vi "Przeliczanie kąta na azymut.vi"(4 "Kąt [stoponie]":dbl) -> (1 "Azymut [stopnie]":dbl)   [LabVIEW 2015, in "Biblioteka moduł map v3.lvlib" / "Matematyczne.lvlib"]
uses:
  Matematyczne.lvlib
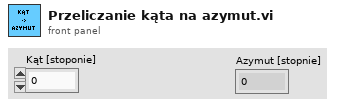
[diagram p1: front panel]
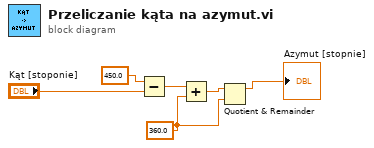
[diagram p0: block diagram]
diagram:
  w4 = 360.0 ("y")
  n1 = Subtract(x=450.0, y="Kąt [stoponie]") -> (x-y=w2:dbl)
  n2 = Add(x=w2, y=w4) -> (x+y=w5:dbl)
  n3 = Quotient & Remainder(x=w5, y=w4) -> (x-y*floor(x/y)=→"Azymut [stopnie]":dbl)  [unwired: 1 out]
